vi "CSDB_Config.delete Data.vi"(2 "InstanceID":string, 5 "error in (no error)":errorcluster) -> (19 "error out":errorcluster)   [LabVIEW 2014, in "CSDB_Config.lvlib"]
doc: "Deletes data of an instance."
uses:
  CSDB_Config.lvlib
  <vilib>/addons/database/Connection.llb/Conn Execute.vi
  <vilib>/addons/database/Recordset.llb/Rec Destroy - Connection.vi
  <vilib>/addons/database/NI_Database_API.lvlib
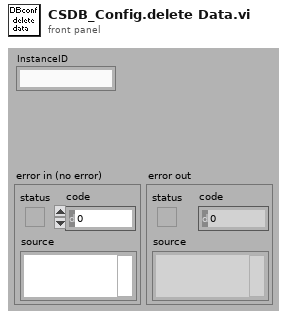
[diagram p1: front panel]
types:
  T1 = typedef "NI_Database_API.lvlib/Conn ObjectReference.ctl" = refnum<k1>
  T2 = typedef "NI_Database_API.lvlib/Rec ObjectReference.ctl" = refnum<k1>
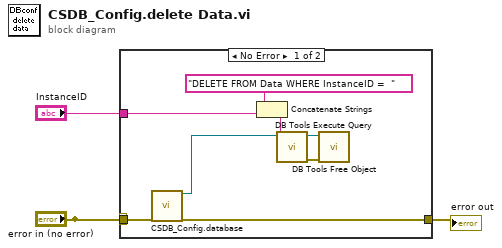
[diagram p0: block diagram]
diagram:
  n1 = case shown="No Error" "error in (no error)" {
    selector: "error in (no error)" -> [_ w12]
    tunnel: "InstanceID" -> [w8 _]
    tunnel: "error in (no error)" -> [w6 _]
    tunnel: [w5 w12] -> w2
    frame No Error {
      n2 = call "CSDB_Config.database.vi"("error in (no error)"=w6) -> ("connectionRef out"=w4:T1, "error out"=w5:errorcluster)  [unwired: 17 in]
      n3 = Concatenate Strings("DELETE FROM Data WHERE InstanceID =  " ("SQL query"), w8) -> (w7:string)
      n4 = call-poly <vilib>:"DB Tools Execute Query.vi"("SQL query"=w7, "connection reference"=w4) -> ("error out"=w10:errorcluster, "recordset reference"=w11:T2)  [unwired: 6 in]
      n5 = call-poly <vilib>:"DB Tools Free Object.vi"("error in (no error)"=w10, "recordset reference"=w11) -> ()  [unwired: 8 in, 2 out]
    }
    frame Error {
    }
  }
  "error out" <- w2
